vi "FPGAinit.vi"(8 "error in":errorcluster, 10 "XAOMsetting":T2(xcontrol), 11 "DIOcluster":T1) -> (0 "error out":errorcluster)   [LabVIEW 2019]
uses:
  controls/xAOMSettings/XAOMsetting.xctl
  <vilib>/Utility/error.llb/Error Cluster From Error Code.vi
  <vilib>/rvi/errors/niLvFpgaAdjustHostInterfaceError.vi
  <vilib>/rvi/interface/nirviReadWriteControl/nirviReadWriteControl.xnode
  NiFpgaLv.dll
  <vilib>/rvi/interface/Simulation/niFpgaSimulationCallBeginRW.vi
panel:
  in  "Bin length /ms":dbl=100.0
  in  "Controller output range":T3={"Output high"=721.0, "Output low"=0.0}
  in  "PID gains":T4={"Proportional gain Kc"=0.01171875, "Integral time Ti [sec]"=0.01953125, "Derivative time Td [sec]"=0.0} {"Integral time Ti [sec]" format="%_6g"}
  # "MW7"
  # "MW8"
  # "XM"
  # "RF"
  # "XR"
  # "AOM"
  # "EOM"
  # "MW"
  # "MW1"
  # "MW2"
  # "MW3"
  # "MW4"
  # "MW5"
  # "MW6"
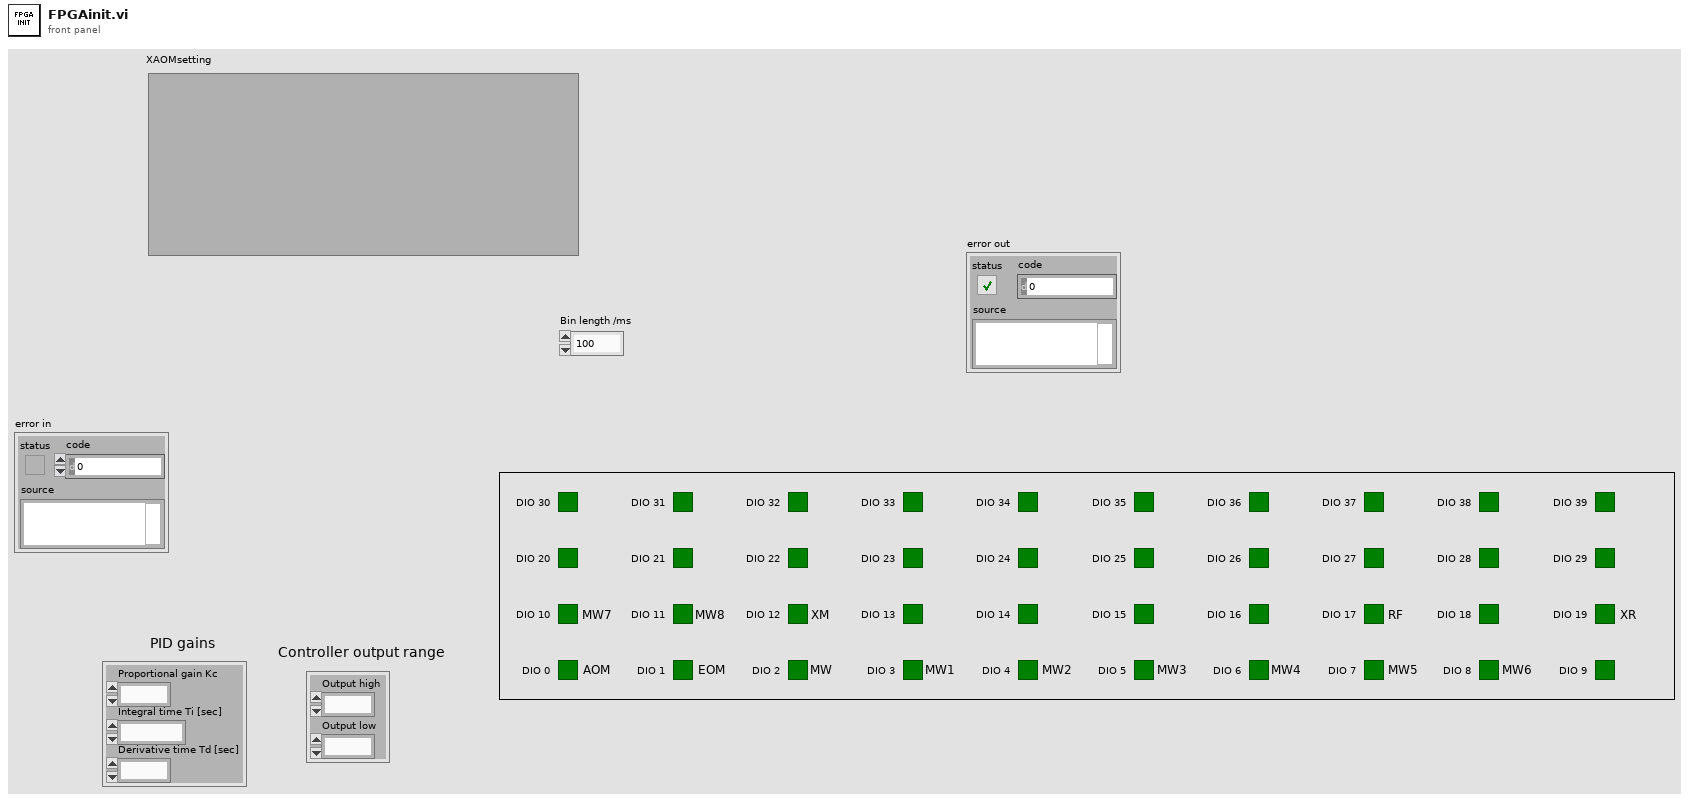
[diagram p1: front panel]
types:
  T1 = cluster{"DIO 0":bool, "DIO 1":bool, "DIO 2":bool, "DIO 3":bool, "DIO 4":bool, "DIO 5":bool, "DIO 6":bool, "DIO 7":bool, "DIO 8":bool, "DIO 9":bool, "DIO 10":bool, "DIO 11":bool, "DIO 12":bool, "DIO 13":bool, "DIO 14":bool, "DIO 15":bool, "DIO 16":bool, "DIO 17":bool, "DIO 18":bool, "DIO 19":bool, "DIO 20":bool, "DIO 21":bool, "DIO 22":bool, "DIO 23":bool, "DIO 24":bool, "DIO 25":bool, "DIO 26":bool, "DIO 27":bool, "DIO 28":bool, "DIO 29":bool, "DIO 30":bool, "DIO 31":bool, "DIO 32":bool, "DIO 33":bool, "DIO 34":bool, "DIO 35":bool, "DIO 36":bool, "DIO 37":bool, "DIO 38":bool, "DIO 39":bool}
  T2 = cluster{"HighPowerNum":dbl, "LowPowerNum":dbl, "PIDnum":dbl, "DeltaFreq":dbl, "BaseFreq":dbl, "AOMout":dbl, "ButtonSelected":enum16{"PID", "Low", "High"}, "AO3":bool}
  T3 = cluster{"Output high":fxp<+/-,16,16>, "Output low":fxp<+/-,16,16>}
  T4 = cluster{"Proportional gain Kc":fxp<+/-,16,8>, "Integral time Ti [sec]":fxp<+/-,16,8>, "Derivative time Td [sec]":fxp<+/-,16,8>}
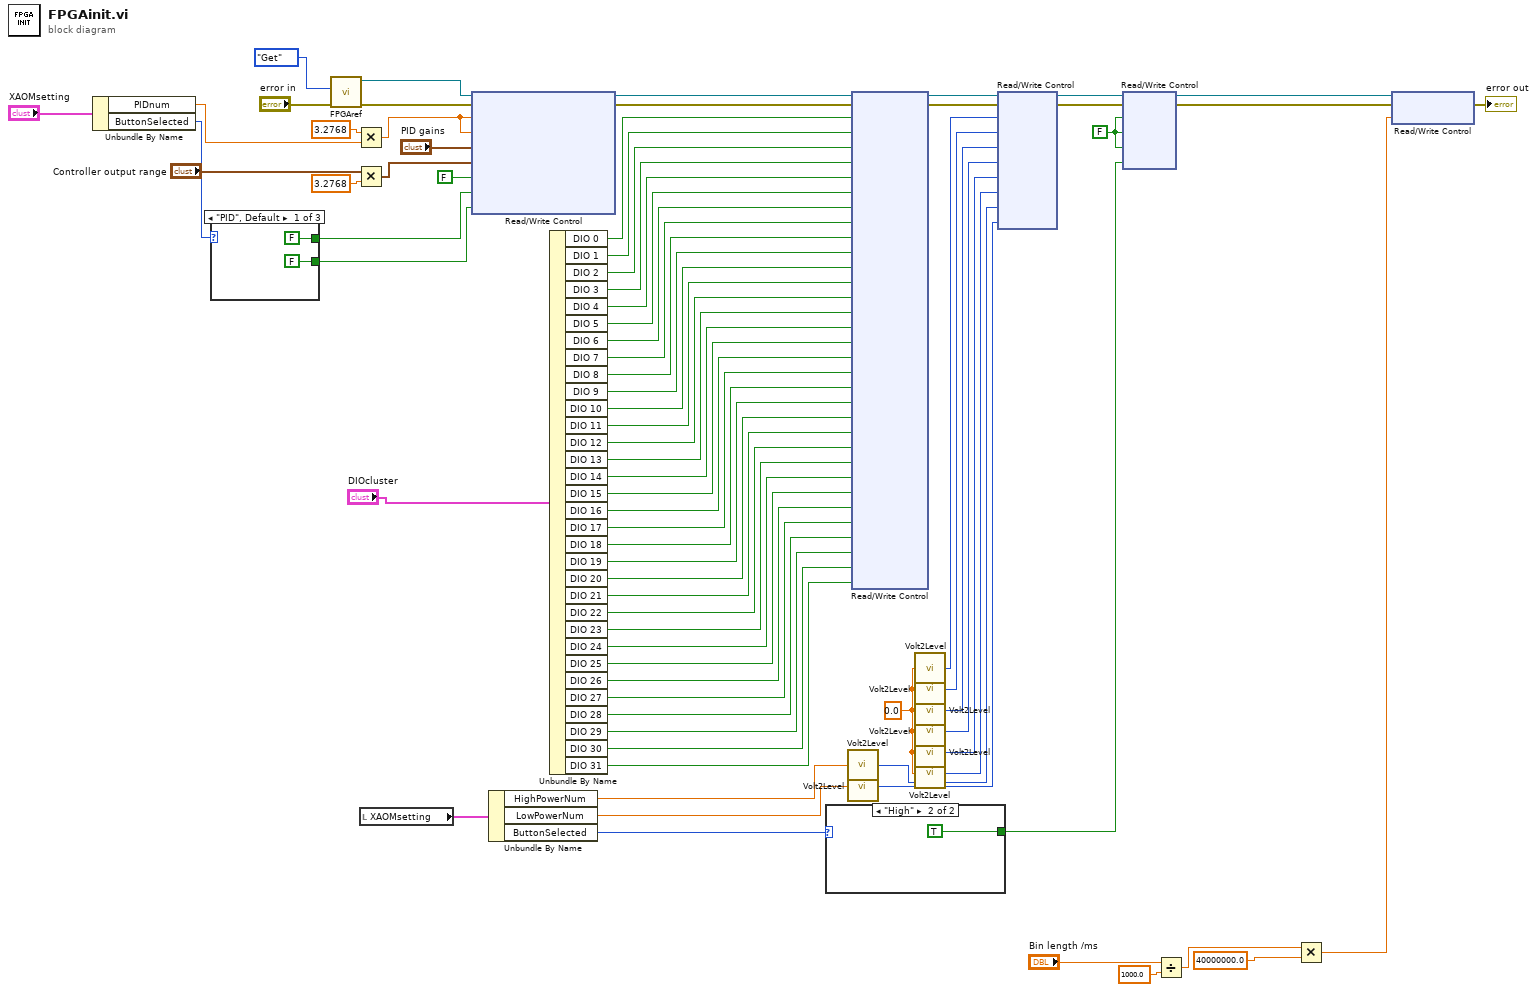
[diagram p0: block diagram]
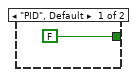
[diagram p2: hidden frame]
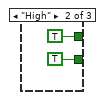
[diagram p3: hidden frame]
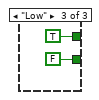
[diagram p4: hidden frame]
diagram:
  w26 = FALSE ("AO1")
  w19 = 0.0 ("voltage /V")
  n1 = Unbundle By Name("XAOMsetting") -> ("PIDnum"=w62:dbl, "ButtonSelected"=w8:enum16{"PID", "Low", "High"})
  n2 = case shown="\"PID\", Default" w8 {
    tunnel: [FALSE TRUE TRUE ("Reinitialise controller")] -> w7
    tunnel: [FALSE TRUE FALSE] -> w6
    frame "PID", Default {
    }
    frame "High" {
    }
    frame "Low" {
    }
  }
  n3 = call "FPGAref.vi"("error in"="error in", "Enum"=enum16{"Set", "Get"}."Get") -> ("error out"=w76:errorcluster, "FPGA VI Reference Out 2"=w77:refnum<k20>)  [unwired: 4 in]
  n4 = Multiply(x=3.2768, y=w62) -> (x*y=w61:dbl)
  n5 = Multiply(x="Controller output range", y=3.2768) -> (x*y=w65:cluster{"Output high":dbl, "Output low":dbl})
  n6 = local read "XAOMsetting"() -> (w28:T2)
  n7 = xnode "Read/Write Control"("FPGA VI Reference In"=w77, "error in"=w76, "Setpoint (H)"=w61, "Setpoint (L)"=w61, "PID gains"="PID gains", "Controller output range"=w65, "Reinitialise controller"=FALSE, "override noise eater?"=w7, "High power"=w6) -> ("FPGA VI Reference Out"=w74:refnum<k20>, "error out"=w73:errorcluster)
  n8 = Unbundle By Name(w28) -> ("HighPowerNum"=w18:dbl, "LowPowerNum"=w17:dbl, "ButtonSelected"=w5:enum16{"PID", "Low", "High"})
  n9 = Unbundle By Name("DIOcluster") -> ("DIO 0"=w60:bool, "DIO 1"=w59:bool, "DIO 2"=w58:bool, "DIO 3"=w57:bool, "DIO 4"=w56:bool, "DIO 5"=w55:bool, "DIO 6"=w54:bool, "DIO 7"=w53:bool, "DIO 8"=w52:bool, "DIO 9"=w51:bool, "DIO 10"=w50:bool, "DIO 11"=w49:bool, "DIO 12"=w48:bool, "DIO 13"=w47:bool, "DIO 14"=w46:bool, "DIO 15"=w45:bool, "DIO 16"=w44:bool, "DIO 17"=w43:bool, "DIO 18"=w42:bool, "DIO 19"=w41:bool, "DIO 20"=w40:bool, "DIO 21"=w39:bool, "DIO 22"=w38:bool, "DIO 23"=w37:bool, "DIO 24"=w36:bool, "DIO 25"=w35:bool, "DIO 26"=w34:bool, "DIO 27"=w33:bool, "DIO 28"=w32:bool, "DIO 29"=w31:bool, "DIO 30"=w30:bool, "DIO 31"=w29:bool)
  n10 = case shown="\"High\"" w5 {
    tunnel: [FALSE TRUE] -> w4
    frame "PID", Default {
    }
    frame "High" {
    }
  }
  n11 = call "Volt2Level.vi"("voltage /V"=w18) -> ("level"=w11:i16)
  n12 = call "Volt2Level.vi"("voltage /V"=w17) -> ("level"=w10:i16)
  n13 = xnode "Read/Write Control"("FPGA VI Reference In"=w74, "error in"=w73, "AOM"=w60, "EOM"=w59, "Microwave"=w58, "dds/ag"=w57, "DIO4"=w56, "DIO5"=w55, "DIO6"=w54, "DIO7"=w53, "DIO8"=w52, "DIO9"=w51, "DIO10"=w50, "DIO11"=w49, "D12"=w48, "D13"=w47, "D14"=w46, "D15"=w45, "D16"=w44, "D17"=w43, "D18"=w42, "D19"=w41, "D20"=w40, "D21"=w39, "D22"=w38, "D23"=w37, "D24"=w36, "D25"=w35, "D26"=w34, "D27"=w33, "D28"=w32, "D29"=w31, "D30"=w30, "D31"=w29) -> ("FPGA VI Reference Out"=w72:refnum<k20>, "error out"=w71:errorcluster)
  n14 = call "Volt2Level.vi"("voltage /V"=w19) -> ("level"=w27:i16)
  n15 = call "Volt2Level.vi"("voltage /V"=w19) -> ("level"=w16:i16)
  n16 = call "Volt2Level.vi"("voltage /V"=w19) -> ("level"=w15:i16)
  n17 = call "Volt2Level.vi"("voltage /V"=w19) -> ("level"=w14:i16)
  n18 = call "Volt2Level.vi"("voltage /V"=w19) -> ("level"=w13:i16)
  n19 = call "Volt2Level.vi"("voltage /V"=w19) -> ("level"=w12:i16)
  n20 = xnode "Read/Write Control"("FPGA VI Reference In"=w72, "error in"=w71, "AO1 on"=w27, "AO1 off"=w16, "AO2 on"=w15, "AO2 off"=w14, "AO3 on"=w13, "AO3 off"=w12, "AO4 on"=w11, "AO4 off"=w10) -> ("FPGA VI Reference Out"=w70:refnum<k20>, "error out"=w69:errorcluster)
  n21 = xnode "Read/Write Control"("FPGA VI Reference In"=w70, "error in"=w69, "AO1"=w26, "AO2"=w26, "AO3"=w26, "AO4"=w4) -> ("FPGA VI Reference Out"=w1:refnum<k20>, "error out"=w2:errorcluster)
  n22 = Divide(x="Bin length /ms", y=1000.0) -> (x/y=w23:dbl)
  n23 = Multiply(x=w23, y=40000000.0) -> (x*y=w21:dbl)
  n24 = xnode "Read/Write Control"("FPGA VI Reference In"=w1, "error in"=w2, "ticks per bin"=w21) -> ("error out"=→"error out":errorcluster)  [unwired: 1 out]
